vi "Exercise 10.1_Answer_Local Variables.vi"() -> ()   [LabVIEW 2010]
uses:
  <vilib>/Analysis/NI_AALBase.lvlib
  <vilib>/Analysis/3filter.llb/Bessel Filter (DBL).vi
panel:
  out "# Data Processed":i32
  in  "stop 2":bool
  out "Missed Data":i32
  out "Consumer Loop Rate (Hz)":u32
  out "Processed Data":dbl[][](graph)
  in  "stop":bool
  out "Raw Data":dbl[][](graph)
  out "Producer Loop Rate (Hz)":u32
  out "# Data Produced":i32
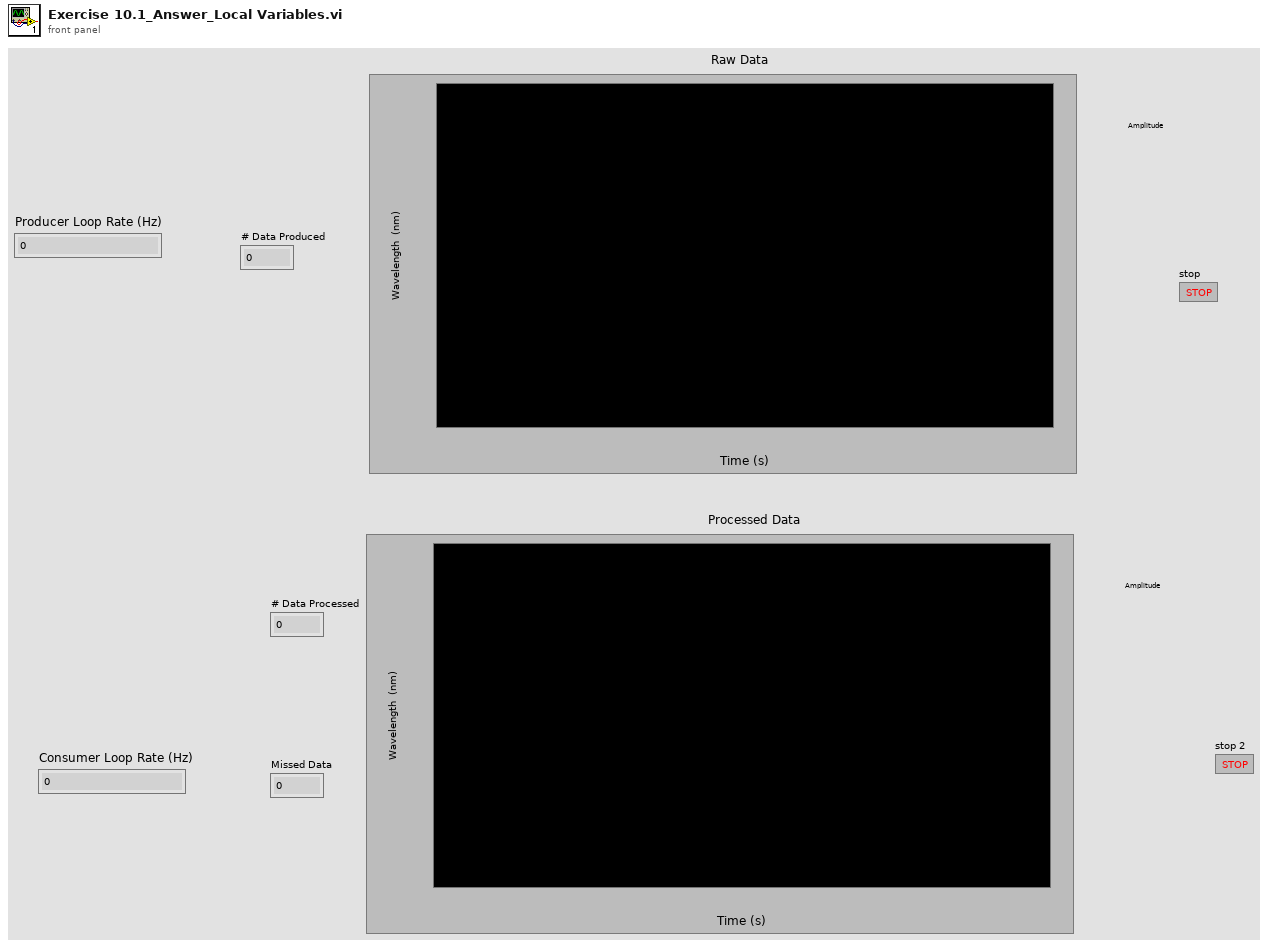
[diagram p1: front panel]
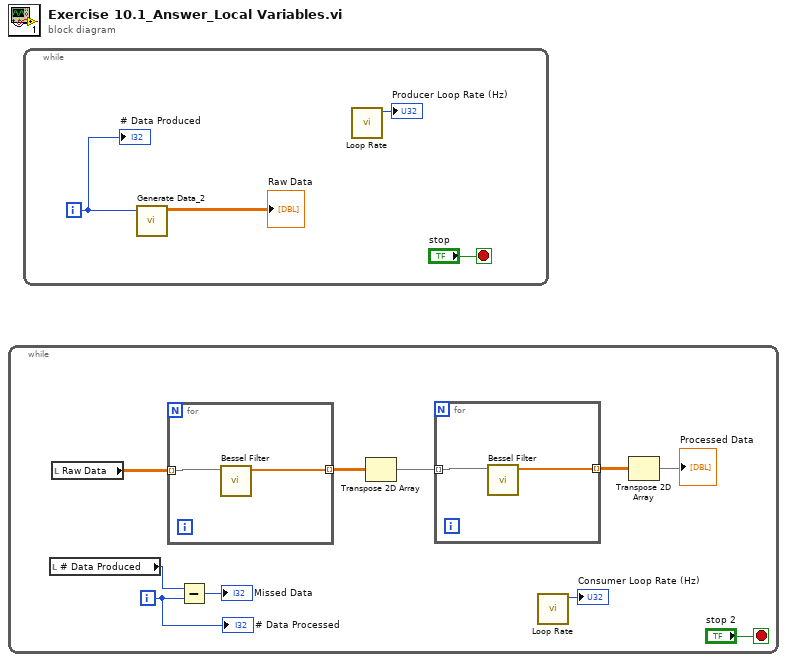
[diagram p0: block diagram]
diagram:
  n1 = while {
    i -> [w3]
    stop <- "stop 2" stop-if-true
    n2 = local read "# Data Produced"() -> (w4:i32)
    n3 = local read "Raw Data"() -> (w10:dbl[][])
    n4 = for {
      tunnel: w10 -> [w14] mode=indexing
      tunnel: [w13] -> w9 mode=indexing
      n5 = call-poly <vilib>:"Bessel Filter.vi"("X"=w14) -> ("Filtered X"=w13:dbl[])  [unwired: 7 in, 1 out]
    }
    n6 = Subtract(x=w4, y=w3) -> (x-y=→"Missed Data":i32)
    n7 = Transpose 2D Array(2D array=w9) -> (transposed array=w8:dbl[][])
    n8 = for {
      tunnel: w8 -> [w12] mode=indexing
      tunnel: [w11] -> w7 mode=indexing
      n9 = call-poly <vilib>:"Bessel Filter.vi"("X"=w12) -> ("Filtered X"=w11:dbl[])  [unwired: 7 in, 1 out]
    }
    n10 = call "Loop Rate.vi"() -> ("Loop Rate (Hz)"=→"Consumer Loop Rate (Hz)":u32)  [unwired: 11 in]
    n11 = Transpose 2D Array(2D array=w7) -> (transposed array=→"Processed Data":dbl[][])
    "# Data Processed" <- w3
  }
  n12 = while {
    i -> [w18]
    stop <- "stop" stop-if-true
    n13 = call "Generate Data_2.vi"("Input"=w18) -> ("Array out"=→"Raw Data":dbl[][])  [unwired: 10 in]
    n14 = call "Loop Rate.vi"() -> ("Loop Rate (Hz)"=→"Producer Loop Rate (Hz)":u32)  [unwired: 11 in]
    "# Data Produced" <- w18
  }
